vi "Parse Boolean Array.vi"(7 "Polling Data Input":T1, 8 "error in (no error)":errorcluster, 11 "Bool Array Input":bool[](array[boolean])) -> (0 "error out":errorcluster, 3 "output cluster":T1)   [LabVIEW 2018]
uses:
  Ctls/DisplayIndicator.ctl
  Ctls/MotroConfigData.ctl
  Ctls/MotorConfig.ctl
  Ctls/MagType.ctl
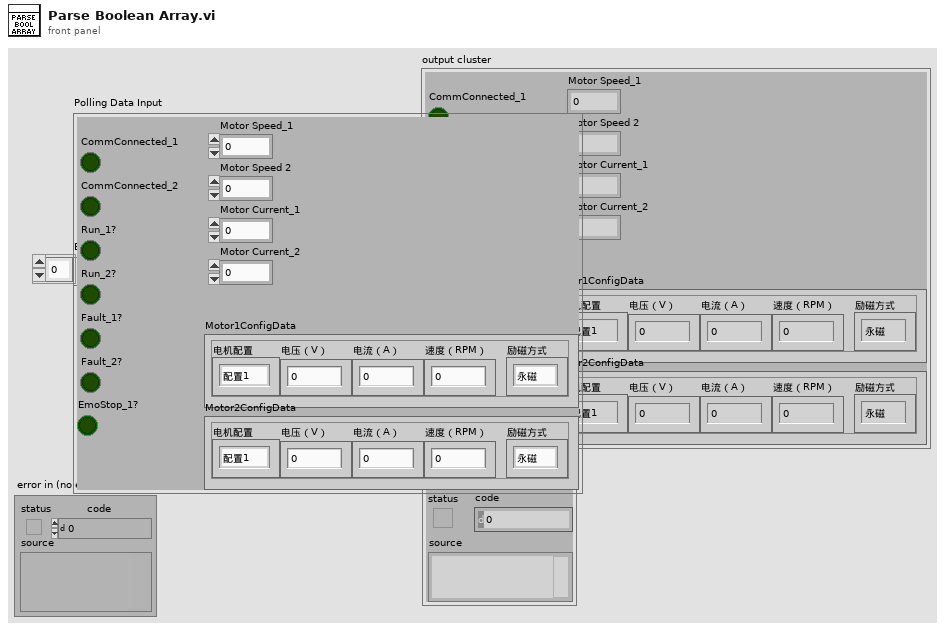
[diagram p1: front panel]
types:
  T1 = typedef "DisplayIndicator.ctl" = cluster{"CommConnected_1":bool, "Run_1?":bool, "Fault_1?":bool, "CommConnected_2":bool, "Run_2?":bool, "Fault_2?":bool, "Motor Speed 2":sgl, "Motor Speed_1":sgl, "Motor Current_1":sgl, "Motor Current_2":sgl, "Motor1ConfigData":T2, "Motor2ConfigData":T2, "EmoStop_1?":bool}
  T2 = typedef "MotroConfigData.ctl" = cluster{"电机配置":T3, "电压（V）":dbl, "电流（A）":dbl, "速度（RPM）":dbl, "励磁方式":T4}
  T3 = typedef "MotorConfig.ctl" = enum16{"配置1", "配置2", "配置3", "配置4"}
  T4 = typedef "MagType.ctl" = enum16{"永磁", "励磁"}
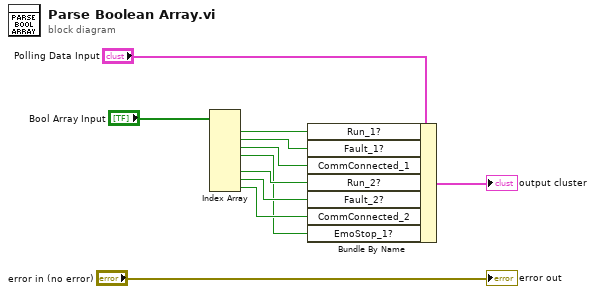
[diagram p0: block diagram]
diagram:
  n1 = Index Array(array="Bool Array Input") -> (element #1=w10:bool, element #2=w9:bool, element #3=w8:bool, element #4=w1:bool, element #6=w7:bool, element #7=w6:bool, element #8=w5:bool)  [unwired: 8 in, 1 out]
  n2 = Bundle By Name(cluster="Polling Data Input", "Run_1?"=w10, "Fault_1?"=w9, "CommConnected_1"=w8, "Run_2?"=w7, "Fault_2?"=w6, "CommConnected_2"=w5, "EmoStop_1?"=w1) -> (→"output cluster":T1)
  "error out" <- "error in (no error)"
